vi "RichToFlatcif_plugincore_FutureTimeEvent.vi"(5 "OutputClusterType":T1, 11 "InputCluster":T2) -> (3 "OutputCluster":T1)   [LabVIEW 2021, in "CIF_Plugin_Core_server.lvlib"]
uses:
  CIF_Plugin_Core_server.lvlib
  cif_plugincore_FutureTimeEvent.ctl
  cif_plugincore_FutureTimeEvent_Flat.ctl
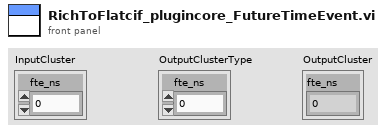
[diagram p1: front panel]
types:
  T1 = typedef "CIF_Plugin_Core_server.lvlib/cif_plugincore_FutureTimeEvent_Flat.ctl" = cluster{"fte_ns":u64}
  T2 = typedef "CIF_Plugin_Core_server.lvlib/cif_plugincore_FutureTimeEvent.ctl" = cluster{"fte_ns":u64}
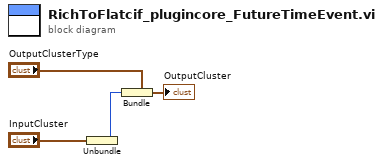
[diagram p0: block diagram]
diagram:
  n1 = Unbundle "Unbundle"("InputCluster") -> ("fte_ns"=w1:u64)
  n2 = Bundle "Bundle"(cluster="OutputClusterType", "fte_ns"=w1) -> (→"OutputCluster":T1)
